vi "fil_device_cal_table.vi"(8 "error_in":errorcluster, 9 "income_table":sgl[][](array[numeric]), 10 "DC":dbl[](array[numeric]), 11 "RMS":dbl[](array[numeric])) -> (0 "error_out":errorcluster, 3 "result_table":sgl[][](array[numeric]))   [LabVIEW 2017]
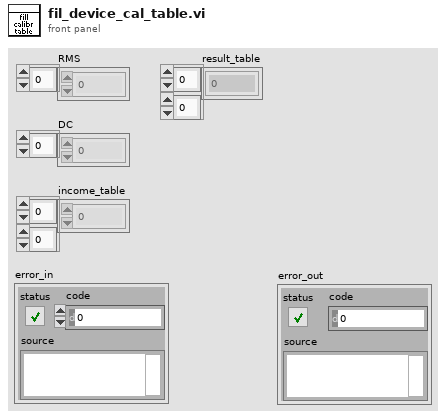
[diagram p1: front panel]
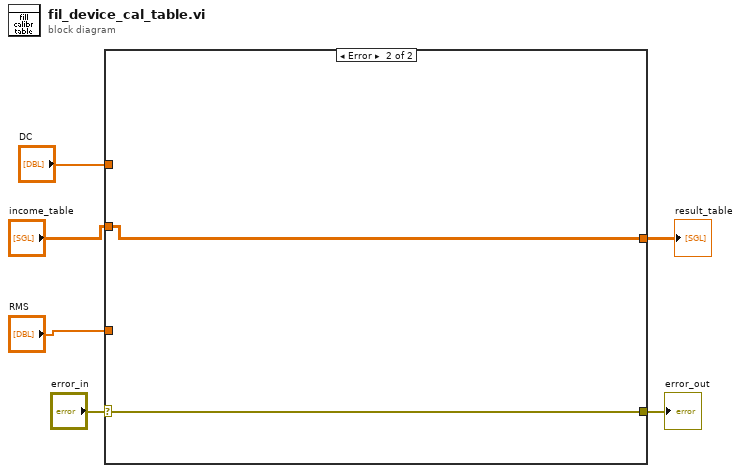
[diagram p0: block diagram]
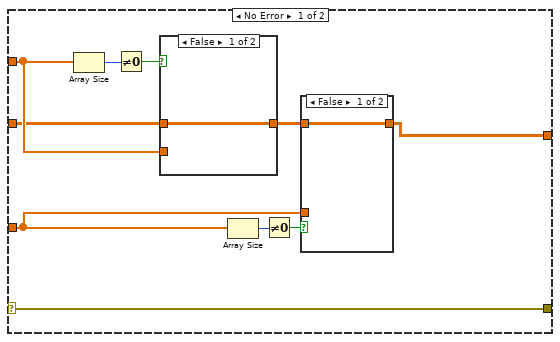
[diagram p2: hidden frame]
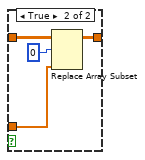
[diagram p3: hidden frame]
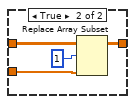
[diagram p4: hidden frame]
diagram:
  n1 = case shown="Error" "error_in" {
    selector: "error_in" -> [w7 w27]
    tunnel: "DC" -> [w11 _]
    tunnel: "income_table" -> [w10 w28]
    tunnel: "RMS" -> [w9 _]
    tunnel: [w8 w28] -> w3
    tunnel: [w7 w27] -> w2
    frame No Error {
      n2 = Array Size(array=w11) -> (size(s)=w15:i32)
      n3 = Not Equal To 0?(x=w15) -> (x != 0?=w14:bool)
      n4 = case shown="False" w14 {
        tunnel: w11 -> [_ w26]
        tunnel: [w22 w25] -> w16
        tunnel: w10 -> [w22 w23]
        frame False {
        }
        frame True {
          n5 = Replace Array Subset(array=w23, new element=w26, index (row)=1) -> (w25:sgl[][])  [unwired: 1 in]
        }
      }
      n6 = Array Size(array=w9) -> (size(s)=w13:i32)
      n7 = Not Equal To 0?(x=w13) -> (x != 0?=w12:bool)
      n8 = case shown="False" w12 {
        tunnel: w9 -> [_ w21]
        tunnel: [w17 w19] -> w8
        tunnel: w16 -> [w17 w18]
        frame False {
        }
        frame True {
          n9 = Replace Array Subset(array=w18, new element=w21, index (row)=0) -> (w19:sgl[][])  [unwired: 1 in]
        }
      }
    }
    frame Error {
    }
  }
  "result_table" <- w3
  "error_out" <- w2
